vi "square_wave_generator.vi"() -> ()   [LabVIEW 2018]
panel:
  out "Waveform Charts":dbl(graph)
  in  "Amplitude":dbl(knob) scale=0.0..10.0
  in  "Frequency(Hz)":dbl(knob) scale=0.0..25.0
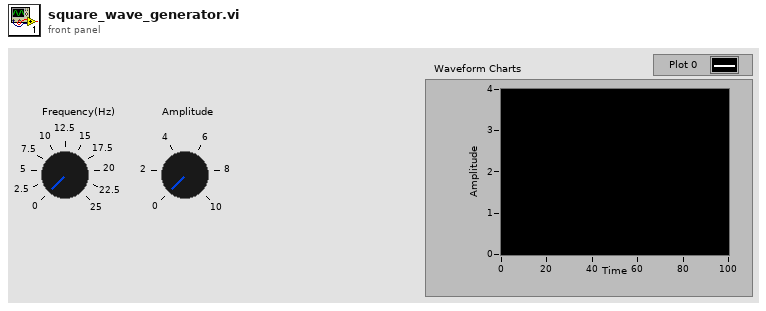
[diagram p1: front panel]
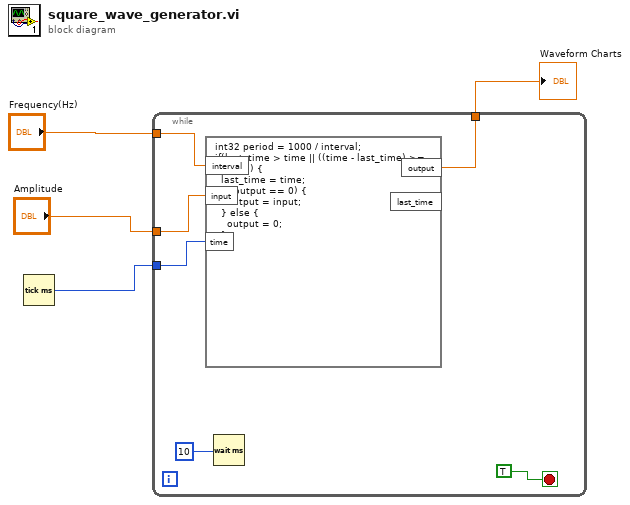
[diagram p0: block diagram]
diagram:
  n1 = Tick Count (ms)() -> (millisecond timer value=w1:u32)
  n2 = while {
    tunnel: [w10] -> w4
    tunnel: "Frequency(Hz)" -> [w9]
    tunnel: "Amplitude" -> [w8]
    tunnel: w1 -> [w7]
    stop <- TRUE stop-if-true
    n3 = formula code="int32 period = 1000 / interval;\nif(last_time > time || ((time - last_time) >= period)) {\n  last_time = time;\n  if (output == 0) {\n    output = input;\n  } else {\n    output = 0;\n  }\n}"("interval"=w9, "input"=w8, "time"=w7) -> ("output"=w10:dbl)  [unwired: 1 out]
    n4 = Wait (ms)(milliseconds to wait=10) -> ()  [unwired: 1 out]
  }
  "Waveform Charts" <- w4
